vi "4PtsTo4Pts.vi"(9 "4PointB":cluster{sgl, sgl}[][](array[cluster]), 10 "4PointA":cluster{"[0]":sgl, "[1]":sgl}[][](array[cluster]), 11 "index":cluster{i32, i32}) -> (3 "A x B":T1)   [LabVIEW 2012]
uses:
  <vilib>/Analysis/Matrix/Datatypes/RealMatrix.ctl
  <vilib>/Analysis/baseanly.llb/Real A x B.vi
  <vilib>/Analysis/baseanly.llb/Real Inverse Matrix.vi
  <vilib>/Analysis/NI_AALBase.lvlib
  <vilib>/Analysis/Matrix/NI_Matrix.lvlib
panel:
  out "appended array":sgl[][](array[numeric])
  out "output array":dbl[][](array[numeric])
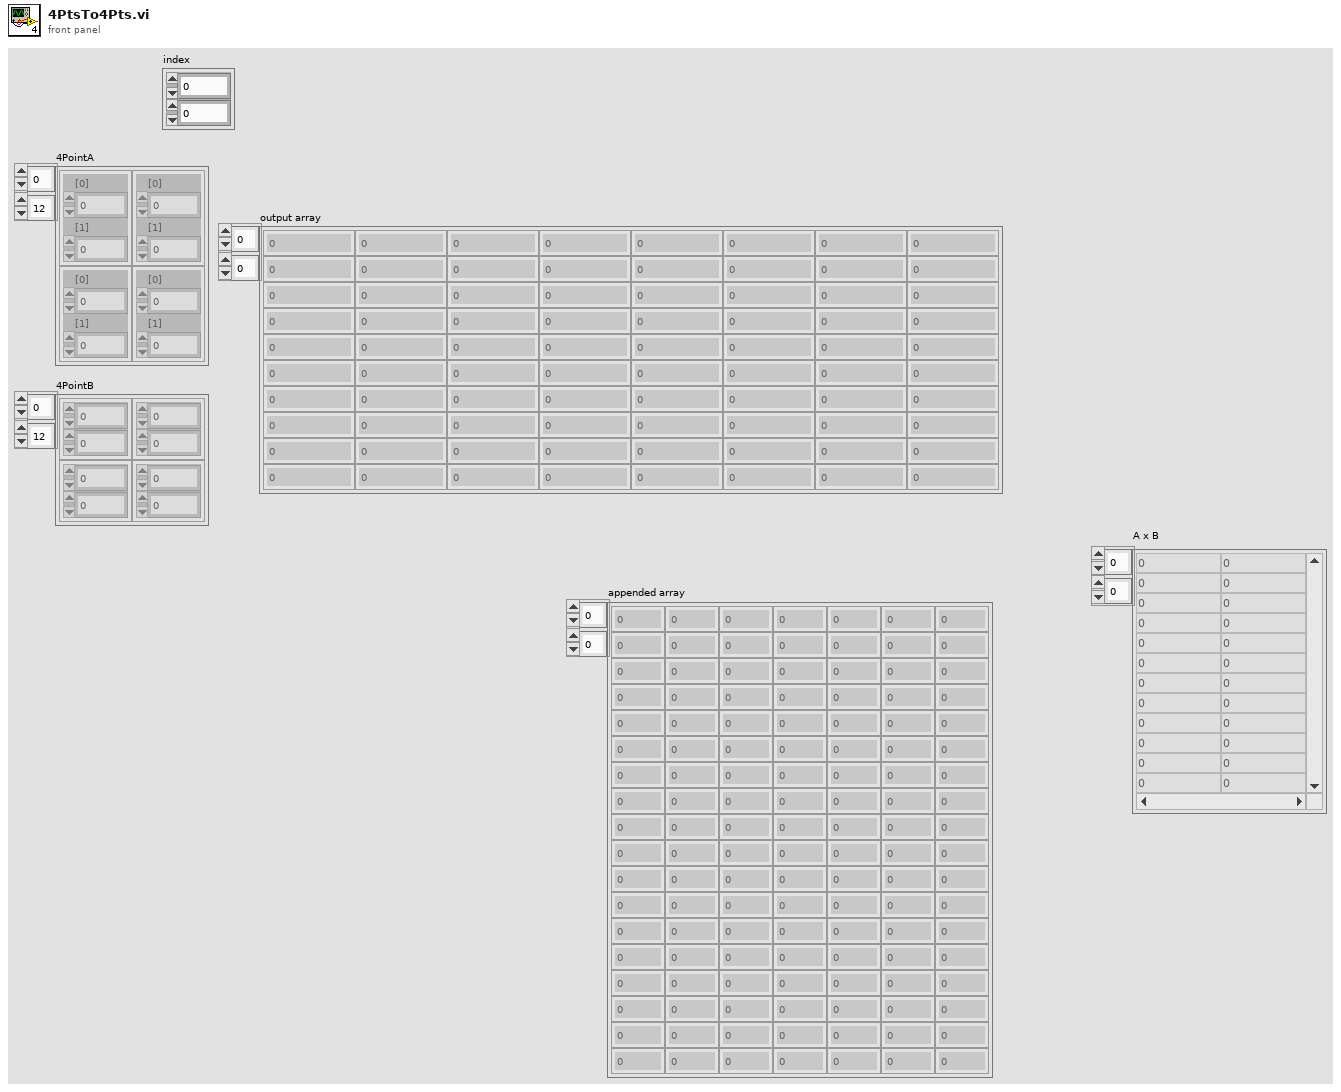
[diagram p1: front panel]
types:
  T1 = typedef "NI_Matrix.lvlib/RealMatrix.ctl" = dbl[][]
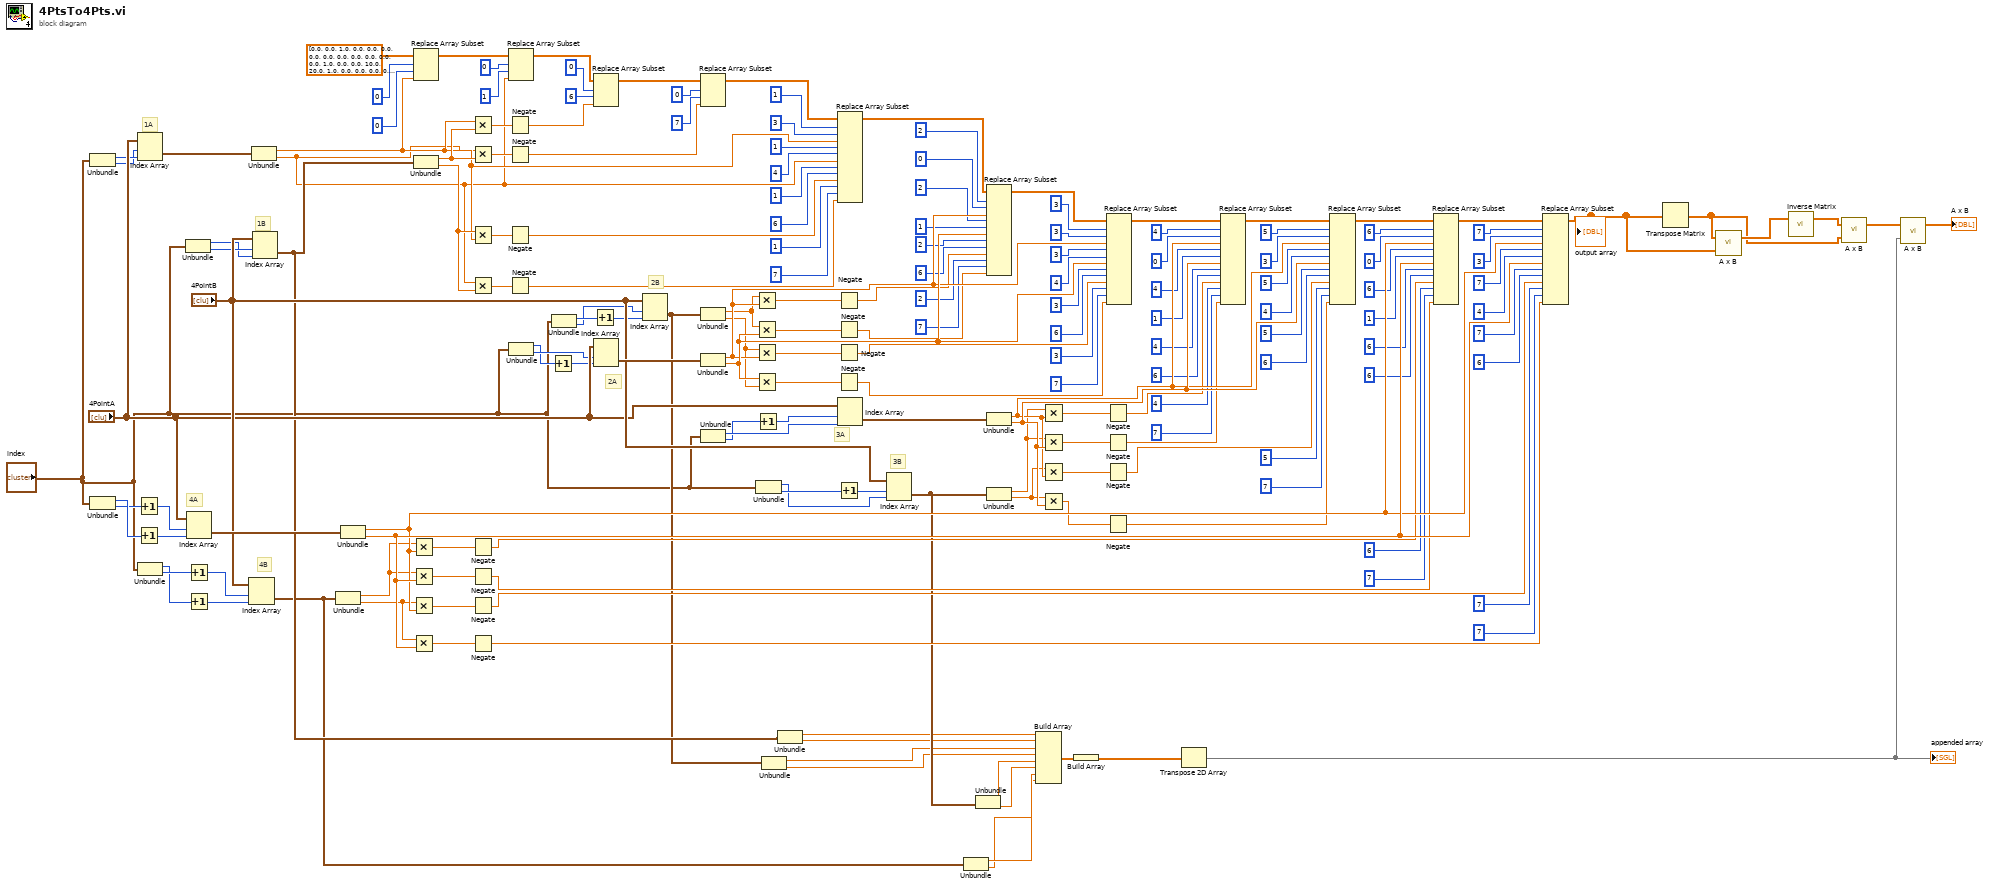
[diagram p0: block diagram]
diagram:
  # "3B"
  # "3A"
  # "2A"
  # "2B"
  # "1B"
  # "4B"
  # "4A"
  # "1A"
  n1 = Unbundle("index") -> (w28:i32, w27:i32)
  n2 = Unbundle("index") -> (w30:i32, w29:i32)
  n3 = Increment(x=w29) -> (x+1=w25:i32)
  n4 = Increment(x=w30) -> (x+1=w26:i32)
  n5 = Index Array(array="4PointA", index (row)=w27, index (col)=w28) -> (element=w53:cluster{"[0]":sgl, "[1]":sgl})
  n6 = Unbundle("index") -> (w44:i32, w45:i32)
  n7 = Unbundle("index") -> (w46:i32, w47:i32)
  n8 = Index Array(array="4PointA", index (row)=w25, index (col)=w26) -> (element=w163:cluster{"[0]":sgl, "[1]":sgl})
  n9 = Increment(x=w45) -> (x+1=w49:i32)
  n10 = Increment(x=w44) -> (x+1=w48:i32)
  n11 = Index Array(array="4PointB", index (row)=w49, index (col)=w48) -> (element=w16:cluster{sgl, sgl})
  n12 = Unbundle(w53) -> ("[0]"=w4:sgl, "[1]"=w3:sgl)
  n13 = Index Array(array="4PointB", index (row)=w47, index (col)=w46) -> (element=w19:cluster{sgl, sgl})
  n14 = Unbundle(w16) -> (w166:sgl, w171:sgl)
  n15 = Unbundle(w163) -> ("[0]"=w172:sgl, "[1]"=w173:sgl)
  n16 = Multiply(x=w166, y=w172) -> (x*y=w164:sgl)
  n17 = Multiply(x=w166, y=w173) -> (x*y=w165:sgl)
  n18 = Multiply(x=w171, y=w172) -> (x*y=w170:sgl)
  n19 = Multiply(x=w171, y=w173) -> (x*y=w169:sgl)
  n20 = Replace Array Subset(array=dbl[][] [[0.0, 0.0, 1.0, 0.0, 0.0, 0.0, 0.0, 0.0], [0.0, 0.0, 0.0, 0.0, 0.0, 1.0, 0.0, 0.0], [10.0, 20.0, 1.0, 0.0, 0.0, 0.0, 0.0, 0.0], [0.0, 0.0, 0.0, 10.0, 20.0, 1.0, -500.0, -1000.0], [41.82, 15.91, 1.0, 0.0, 0.0, 0.0, -2091.0, -795.5], [0.0, 0.0, 0.0, 41.82, 15.91, 1.0, -2091.0, -795.5], [50.0, 0.0, 1.0, 0.0, 0.0, 0.0, -2500.0, 0.0], [0.0, 0.0, 0.0, 50.0, 0.0, 1.0, 0.0, 0.0]], new element=w4, index (row)=0, index (col)=0 ("disabled index (col)")) -> (w61:dbl[][])
  n21 = Unbundle(w19) -> (w75:sgl, w82:sgl)
  n22 = Multiply(x=w4, y=w75) -> (x*y=w65:sgl)
  n23 = Multiply(x=w3, y=w75) -> (x*y=w66:sgl)
  n24 = Multiply(x=w82, y=w4) -> (x*y=w76:sgl)
  n25 = Multiply(x=w3, y=w82) -> (x*y=w80:sgl)
  n26 = Negate(x=w164) -> (-x=w167:sgl)
  n27 = Negate(x=w165) -> (-x=w168:sgl)
  n28 = Negate(x=w170) -> (-x=w174:sgl)
  n29 = Negate(x=w169) -> (-x=w175:sgl)
  n30 = Negate(x=w65) -> (-x=w92:sgl)
  n31 = Negate(x=w66) -> (-x=w67:sgl)
  n32 = Negate(x=w76) -> (-x=w77:sgl)
  n33 = Negate(x=w80) -> (-x=w81:sgl)
  n34 = Replace Array Subset(array=w61, new element=w3, index (row)=0, index (col)=1 ("disabled index (col)")) -> (w62:dbl[][])
  n35 = Unbundle("index") -> (w31:i32, w33:i32)
  n36 = Increment(x=w31) -> (x+1=w32:i32)
  n37 = Unbundle("index") -> (w43:i32, w41:i32)
  n38 = Increment(x=w43) -> (x+1=w42:i32)
  n39 = Replace Array Subset(array=w62, new element=w92, index (row)=0, index (col)=6 ("disabled index (col)")) -> (w63:dbl[][])
  n40 = Index Array(array="4PointA", index (row)=w33, index (col)=w32) -> (element=w64:cluster{"[0]":sgl, "[1]":sgl})
  n41 = Index Array(array="4PointB", index (row)=w41, index (col)=w42) -> (element=w18:cluster{sgl, sgl})
  n42 = Replace Array Subset(array=w63, new element=w67, index (row)=0, index (col)=7 ("disabled index (col)")) -> (w68:dbl[][])
  n43 = Unbundle(w18) -> (w95:sgl, w109:sgl)
  n44 = Unbundle(w64) -> ("[0]"=w110:sgl, "[1]"=w111:sgl)
  n45 = Unbundle("index") -> (w36:i32, w34:i32)
  n46 = Multiply(x=w95, y=w110) -> (x*y=w93:sgl)
  n47 = Multiply(x=w95, y=w111) -> (x*y=w96:sgl)
  n48 = Multiply(x=w109, y=w110) -> (x*y=w108:sgl)
  n49 = Multiply(x=w111, y=w109) -> (x*y=w107:sgl)
  n50 = Increment(x=w34) -> (x+1=w35:i32)
  n51 = Unbundle("index") -> (w38:i32, w40:i32)
  n52 = Unbundle(w18) -> (w13:sgl, w12:sgl)
  n53 = Unbundle(w19) -> (w15:sgl, w14:sgl)
  n54 = Negate(x=w93) -> (-x=w94:sgl)
  n55 = Negate(x=w96) -> (-x=w97:sgl)
  n56 = Negate(x=w108) -> (-x=w112:sgl)
  n57 = Negate(x=w107) -> (-x=w113:sgl)
  n58 = Increment(x=w40) -> (x+1=w39:i32)
  n59 = Replace Array Subset(array=w68, new element #1=w4, index (row) #1=1 ("index (row)"), index (col) #1=3 ("disabled index (col)"), new element #2=w3, index (row) #2=1 ("index (row)"), index (col) #2=4 ("disabled index (col)"), new element #3=w77, index (row) #3=1 ("index (row)"), index (col) #3=6 ("disabled index (col)"), new element #4=w81, index (row) #4=1 ("index (row)"), index (col) #4=7 ("disabled index (col)")) -> (w83:dbl[][])
  n60 = Index Array(array="4PointA", index (row)=w35, index (col)=w36) -> (element=w123:cluster{"[0]":sgl, "[1]":sgl})
  n61 = Index Array(array="4PointB", index (row)=w39, index (col)=w38) -> (element=w17:cluster{sgl, sgl})
  n62 = Unbundle(w16) -> (w9:sgl, w8:sgl)
  n63 = Unbundle(w17) -> (w11:sgl, w10:sgl)
  n64 = Replace Array Subset(array=w83, new element #1=w110, index (row) #1=2 ("index (row)"), index (col) #1=0 ("disabled index (col)"), new element #2=w111, index (row) #2=2 ("index (row)"), index (col) #2=1 ("disabled index (col)"), new element #3=w94, index (row) #3=2 ("index (row)"), index (col) #3=6 ("disabled index (col)"), new element #4=w97, index (row) #4=2 ("index (row)"), index (col) #4=7 ("disabled index (col)")) -> (w98:dbl[][])
  n65 = Unbundle(w123) -> ("[0]"=w141:sgl, "[1]"=w142:sgl)
  n66 = Unbundle(w17) -> (w126:sgl, w140:sgl)
  n67 = Build Array(w15, w14, w13, w12, w11, w10, w9, w8) -> (w7:sgl[])
  n68 = Multiply(x=w126, y=w141) -> (x*y=w124:sgl)
  n69 = Multiply(x=w126, y=w142) -> (x*y=w125:sgl)
  n70 = Multiply(x=w140, y=w141) -> (x*y=w139:sgl)
  n71 = Multiply(x=w140, y=w142) -> (x*y=w138:sgl)
  n72 = Build Array(w7) -> (w6:sgl[][])
  n73 = Negate(x=w124) -> (-x=w127:sgl)
  n74 = Negate(x=w125) -> (-x=w128:sgl)
  n75 = Negate(x=w139) -> (-x=w143:sgl)
  n76 = Negate(x=w138) -> (-x=w144:sgl)
  n77 = Replace Array Subset(array=w98, new element #1=w110, index (row) #1=3 ("index (row)"), index (col) #1=3 ("disabled index (col)"), new element #2=w111, index (row) #2=3 ("index (row)"), index (col) #2=4 ("disabled index (col)"), new element #3=w112, index (row) #3=3 ("index (row)"), index (col) #3=6 ("disabled index (col)"), new element #4=w113, index (row) #4=3 ("index (row)"), index (col) #4=7 ("disabled index (col)")) -> (w114:dbl[][])
  n78 = Transpose 2D Array(2D array=w6) -> (transposed array=w5:sgl[][])
  "appended array" <- w5
  n79 = Replace Array Subset(array=w114, new element #1=w141, index (row) #1=4 ("index (row)"), index (col) #1=0 ("disabled index (col)"), new element #2=w142, index (row) #2=4 ("index (row)"), index (col) #2=1 ("disabled index (col)"), new element #3=w127, index (row) #3=4 ("index (row)"), index (col) #3=6 ("disabled index (col)"), new element #4=w128, index (row) #4=4 ("index (row)"), index (col) #4=7 ("disabled index (col)")) -> (w136:dbl[][])
  n80 = Replace Array Subset(array=w136, new element #1=w141, index (row) #1=5 ("disabled index (row)"), index (col) #1=3 ("disabled index (col)"), new element #2=w142, index (row) #2=5 ("index (row)"), index (col) #2=4 ("disabled index (col)"), new element #3=w143, index (row) #3=5 ("index (row)"), index (col) #3=6 ("disabled index (col)"), new element #4=w144, index (row) #4=5 ("index (row)"), index (col) #4=7 ("disabled index (col)")) -> (w161:dbl[][])
  n81 = Replace Array Subset(array=w161, new element #1=w172, index (row) #1=6 ("index (row)"), index (col) #1=0 ("disabled index (col)"), new element #2=w173, index (row) #2=6 ("index (row)"), index (col) #2=1 ("disabled index (col)"), new element #3=w167, index (row) #3=6 ("index (row)"), index (col) #3=6 ("disabled index (col)"), new element #4=w168, index (row) #4=6 ("index (row)"), index (col) #4=7 ("disabled index (col)")) -> (w162:dbl[][])
  n82 = Replace Array Subset(array=w162, new element #1=w172, index (row) #1=7 ("disabled index (row)"), index (col) #1=3 ("disabled index (col)"), new element #2=w173, index (row) #2=7 ("index (row)"), index (col) #2=4 ("disabled index (col)"), new element #3=w174, index (row) #3=7 ("index (row)"), index (col) #3=6 ("disabled index (col)"), new element #4=w175, index (row) #4=7 ("index (row)"), index (col) #4=7 ("disabled index (col)")) -> (w20:dbl[][])
  "output array" <- w20
  n83 = Transpose Matrix(1:w20) -> (0:w22:dbl[][])
  n84 = call-poly <vilib>:"A x B.vi"("B"=w20, "A"=w22) -> ("A x B"=w24:T1)  [unwired: 1 out]
  n85 = call-poly <vilib>:"Inverse Matrix.vi"("Input Matrix"=w24) -> ("Inverse Matrix"=w23:T1)  [unwired: 1 in, 1 out]
  n86 = call-poly <vilib>:"A x B.vi"("B"=w22, "A"=w23) -> ("A x B"=w21:T1)  [unwired: 1 out]
  n87 = call-poly <vilib>:"A x B.vi"("B"=w5, "A"=w21) -> ("A x B"=→"A x B":T1)  [unwired: 1 out]
